vi "使用状态机的测试程序.vi"   [LabVIEW 2022 SP3]
doc: "本VI是为《我和LabVIEW》一书编写的示例。\n关于本书的介绍请参考网页：\nhttp://ruanqizhen.spaces.live.com/blog/cns!5852D4F797C53FB6!4310.entry"
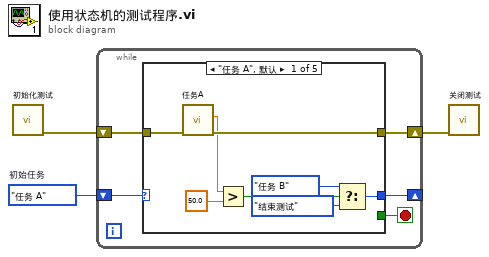
[diagram p0: block diagram]
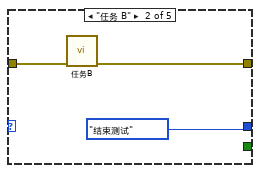
[diagram p2: hidden frame]
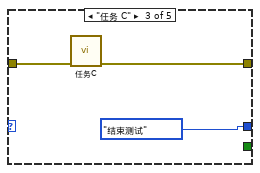
[diagram p3: hidden frame]
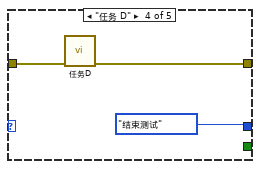
[diagram p4: hidden frame]
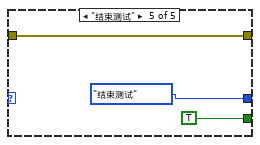
[diagram p5: hidden frame]
diagram:
  w1 = enum16{"任务 A", "任务 B", "任务 C", "任务 D", "结束测试"}."任务 A"  # 初始任务
  n1 = call "初始化测试.vi"() -> ("error out"=w3:errorcluster)  [unwired: 1 in, 10 out]
  n2 = while {
    shift-right: [w6] -> w2
    shift-left: w3 -> [w7]
    shift-right: [w5] -> _
    shift-left: w1 -> [w8]
    stop <- w4 stop-if-true
    n3 = case shown="\"任务 A\", 默认" w8 {
      tunnel: w7 -> [w16 w19 w22 w25 w27]
      tunnel: [w15 w18 w21 w24 w27] -> w6
      tunnel: [w11 enum16{"任务 A", "任务 B", "任务 C", "任务 D", "结束测试"}."结束测试" ("初始任务") enum16{"任务 A", "任务 B", "任务 C", "任务 D", "结束测试"}."结束测试" ("初始任务") enum16{"任务 A", "任务 B", "任务 C", "任务 D", "结束测试"}."结束测试" ("初始任务") enum16{"任务 A", "任务 B", "任务 C", "任务 D", "结束测试"}."结束测试" ("初始任务")] -> w5
      tunnel: [_ _ _ _ TRUE] -> w4
      frame "任务 A", Default {
        n4 = call "任务A.vi"("error in (no error)"=w16) -> ("error out"=w15:errorcluster, "数值"=w14:dbl)  [unwired: 1 in, 8 out]
        n5 = Greater?(x=w14, y=50.0) -> (0:w9:bool)
        n6 = Select(t=enum16{"任务 A", "任务 B", "任务 C", "任务 D", "结束测试"}."任务 B" ("初始任务"), s=w9, f=enum16{"任务 A", "任务 B", "任务 C", "任务 D", "结束测试"}."结束测试" ("初始任务")) -> (s? t:f=w11:enum16{"任务 A", "任务 B", "任务 C", "任务 D", "结束测试"})
      }
      frame "任务 B" {
        n7 = call "任务B.vi"("error in (no error)"=w19) -> ("error out"=w18:errorcluster)  [unwired: 1 in, 9 out]
      }
      frame "任务 C" {
        n8 = call "任务C.vi"("error in (no error)"=w22) -> ("error out"=w21:errorcluster)  [unwired: 1 in, 9 out]
      }
      frame "任务 D" {
        n9 = call "任务D.vi"("error in (no error)"=w25) -> ("error out"=w24:errorcluster)  [unwired: 1 in, 9 out]
      }
      frame "结束测试" {
      }
    }
  }
  n10 = call "关闭测试.vi"("error in (no error)"=w2) -> ()  [unwired: 11 out]
